vi "Ethernet IP Custom Device Initialization VI.vi"(8 "error in (no error)":errorcluster, 10 "Custom XML":string, 11 "Device Item Ref in":T1 format="%.0x") -> (0 "error out":errorcluster, 3 "Device Item Ref out":T1 format="%.0x")   [LabVIEW 2011, in "Ethernet IP Custom Device Custom Device.lvlib"]
uses:
  Ethernet IP Custom Device Custom Device.lvlib
  <vilib>/NI Veristand/Custom Device API/Custom Device Item Ref.ctl
  <vilib>/NI Veristand/Custom Device API/Custom Device Timed Loop Priority.ctl
  <vilib>/NI Veristand/Custom Device API/Custom Device Loop Type.ctl
  Ethernet IP Global Strings.vi
  Ethernet IP Global GUIDs.vi
  <vilib>/NI Veristand/Custom Device API/Set Item Property (String).vi
  <vilib>/NI Veristand/Custom Device API/Set Item Property (I32).vi
  <vilib>/NI Veristand/Custom Device API/Set Item Property (Path).vi
  <vilib>/NI Veristand/Custom Device API/Custom Device API.lvlib
panel:
  in  "Import Info":string="Unconfigured tags are tags that we need to specify if they are inputs or outputs.\n\nAlso provides information about tags that we couldn't import in a successful manner (due to incompatible data types for an example)."
  in  "IO Folder":string="Tags are devided up into an input section and an output section.\n \nPress the \"Input\" section in tree to see tag inputs and press the \"Output\"\nsection to see the tag outputs."
  in  "Description":string="This Custom Device will allow communication with targets that support communications using Logix tag names over Ethernet/IP.  \n\nValid targets include PLCs such as the Rockwell ControlLogix series.\n\nSupported data types in this custom device:\nSINT\nINT\nDINT\nREAL\nBOOL \nSTRING"
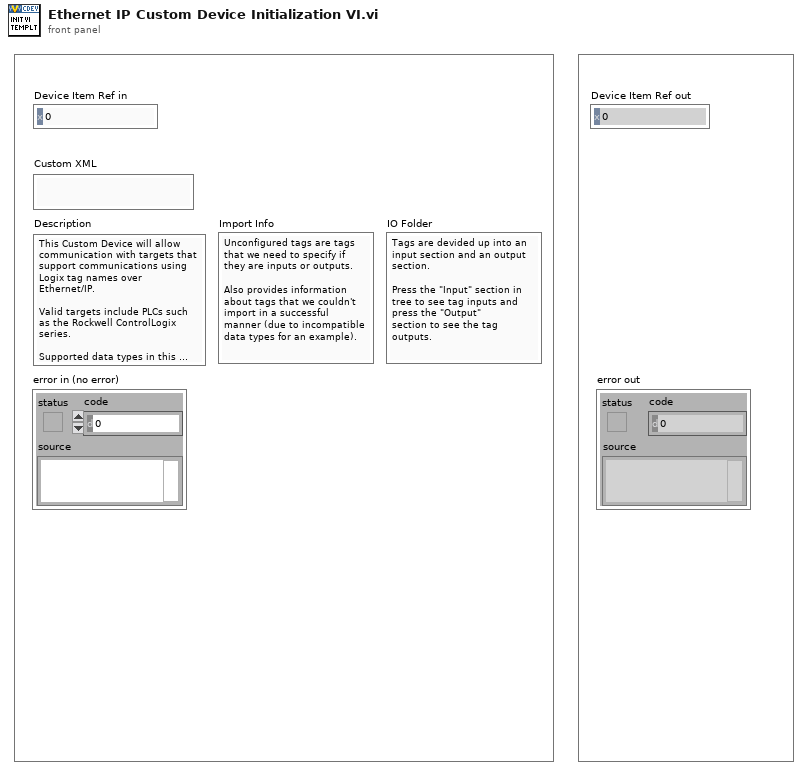
[diagram p1: front panel]
types:
  T1 = typedef "Custom Device API.lvlib/Custom Device Item Ref.ctl" = u64
  T2 = typedef "Custom Device API.lvlib/Custom Device Timed Loop Priority.ctl" = enum32{"Low", "Medium", "High"}
  T3 = typedef "Custom Device API.lvlib/Custom Device Loop Type.ctl" = enum32{"While Loop", "Timed Loop"}
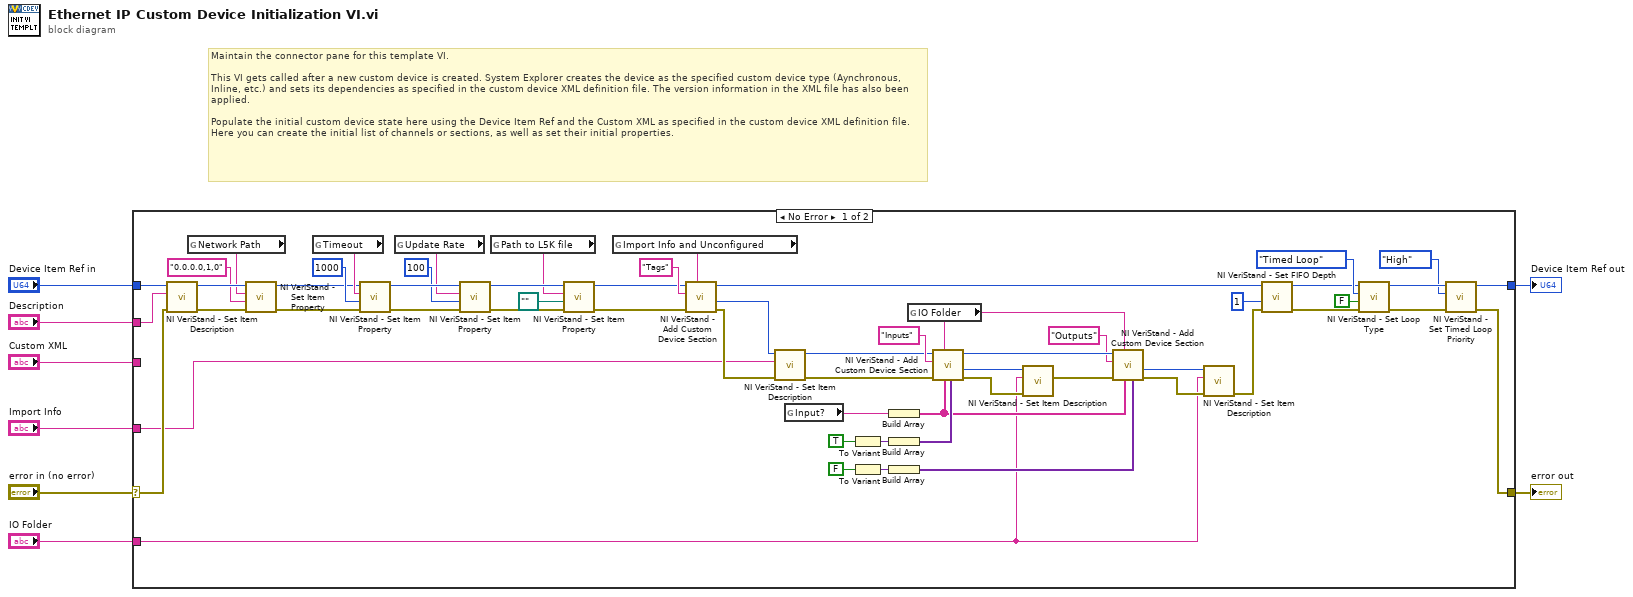
[diagram p0: block diagram]
diagram:
  # "Maintain the connector pane for this template VI.\n\nThis VI gets called after a new custom device is created. System Explorer creates the device as the specified custom device type (Aynchronous, Inline, etc.) and sets its dependencies as specified in the custom device XML definition file. The version information in the XML file has also been applied.\n\nPopulate the initial custom device state here using the Device Item Ref and the Custom XML as specified in the custom device XML definition file. Here you can create the initial list of channels or sections, as well as set their initial properties."
  n1 = case shown="No Error" "error in (no error)" {
    selector: "error in (no error)" -> [w58 w68]
    tunnel: [w9 w68] -> w8
    tunnel: [w12 w67] -> w6
    tunnel: "Device Item Ref in" -> [w63 w67]
    tunnel: "Custom XML" -> [_ _]
    tunnel: "Description" -> [w59 _]
    tunnel: "IO Folder" -> [w19 _]
    tunnel: "Import Info" -> [w18 _]
    frame No Error {
      n2 = call <vilib>:"NI VeriStand - Set Item Description.vi"("error in (no error)"=w58, "Description"=w59, "Item Ref in"=w63) -> ("error out"=w66:errorcluster, "Item Ref out"=w62:T1)  [unwired: 6 in, 1 out]
      n3 = global read "Ethernet IP Global Strings.vi" "Network Path"() -> (w57:string)
      n4 = call-poly <vilib>:"NI VeriStand - Set Item Property.vi"("error in (no error)"=w66, "Value"="0.0.0.0,1,0", "Property Name"=w57, "Item Ref in"=w62) -> ("error out"=w40:errorcluster, "Item Ref out"=w41:T1)  [unwired: 5 in, 1 out]
      n5 = global read "Ethernet IP Global Strings.vi" "Timeout"() -> (w56:string)
      n6 = call-poly <vilib>:"NI VeriStand - Set Item Property.vi"("error in (no error)"=w40, "Value"=1000, "Property Name"=w56, "Item Ref in"=w41) -> ("error out"=w64:errorcluster, "Item Ref out"=w61:T1)  [unwired: 5 in, 1 out]
      n7 = global read "Ethernet IP Global Strings.vi" "Update Rate"() -> (w55:string)
      n8 = call-poly <vilib>:"NI VeriStand - Set Item Property.vi"("error in (no error)"=w64, "Value"=100, "Property Name"=w55, "Item Ref in"=w61) -> ("error out"=w31:errorcluster, "Item Ref out"=w30:T1)  [unwired: 5 in, 1 out]
      n9 = global read "Ethernet IP Global Strings.vi" "Path to L5K file"() -> (w27:string)
      n10 = call-poly <vilib>:"NI VeriStand - Set Item Property.vi"("error in (no error)"=w31, "Value"=path "", "Property Name"=w27, "Item Ref in"=w30) -> ("error out"=w28:errorcluster, "Item Ref out"=w29:T1)  [unwired: 5 in, 1 out]
      n11 = global read "Ethernet IP Global GUIDs.vi" "Import Info and Unconfigured"() -> (w36:string)
      n12 = call <vilib>:"NI VeriStand - Add Custom Device Section.vi"("GUID (Default Section)"=w36, "error in (no error)"=w28, "Section Name"="Tags", "Parent Ref in"=w29) -> ("error out"=w34:errorcluster, "Section Ptr"=w35:T1, "Parent Ref out"=w37:T1)  [unwired: 4 in, 1 out]
      n13 = call <vilib>:"NI VeriStand - Set Item Description.vi"("error in (no error)"=w34, "Description"=w18, "Item Ref in"=w35) -> ("error out"=w33:errorcluster, "Item Ref out"=w32:T1)  [unwired: 6 in, 1 out]
      n14 = global read "Ethernet IP Global Strings.vi" "Input?"() -> (w42:string)
      n15 = To Variant(anything=TRUE) -> (Variant=w47:variant)
      n16 = To Variant(anything=FALSE) -> (Variant=w46:variant)
      n17 = Build Array(w42) -> (w43:string[])
      n18 = Build Array(w47) -> (w45:variant[])
      n19 = Build Array(w46) -> (w44:variant[])
      n20 = global read "Ethernet IP Global GUIDs.vi" "IO Folder"() -> (w50:string)
      n21 = call <vilib>:"NI VeriStand - Add Custom Device Section.vi"("Property Values"=w45, "Property names"=w43, "GUID (Default Section)"=w50, "error in (no error)"=w33, "Section Name"="Inputs", "Parent Ref in"=w32) -> ("error out"=w21:errorcluster, "Section Ptr"=w22:T1, "Parent Ref out"=w60:T1)  [unwired: 2 in, 1 out]
      n22 = call <vilib>:"NI VeriStand - Set Item Description.vi"("error in (no error)"=w21, "Description"=w19, "Item Ref in"=w22) -> ("error out"=w20:errorcluster)  [unwired: 6 in, 2 out]
      n23 = call <vilib>:"NI VeriStand - Add Custom Device Section.vi"("Property Values"=w44, "Property names"=w43, "GUID (Default Section)"=w50, "error in (no error)"=w20, "Section Name"="Outputs", "Parent Ref in"=w60) -> ("error out"=w24:errorcluster, "Section Ptr"=w25:T1)  [unwired: 2 in, 2 out]
      n24 = call <vilib>:"NI VeriStand - Set Item Description.vi"("error in (no error)"=w24, "Description"=w19, "Item Ref in"=w25) -> ("error out"=w23:errorcluster)  [unwired: 6 in, 2 out]
      n25 = call <vilib>:"NI VeriStand - Set FIFO Depth.vi"("error in (no error)"=w23, "Size FIFO Sink (1)"=u32 1 ("Size FIFO Source (1)"), "Device Ref in"=w37) -> ("error out"=w14:errorcluster, "Device Ref out"=w15:T1)  [unwired: 7 in]
      n26 = call <vilib>:"NI VeriStand - Set Loop Type.vi"("error in (no error)"=w14, "Use Device Clock (Timed Loops only)"=FALSE, "Loop type"=Custom_Device_Loop_Type."Timed Loop", "Device Ref in"=w15) -> ("error out"=w10:errorcluster, "Device Ref out"=w13:T1)  [unwired: 6 in]
      n27 = call <vilib>:"NI VeriStand - Set Timed Loop Priority.vi"("error in (no error)"=w10, "Priority"=Custom_Device_Timed_Loop_Priority."High", "Device Ref in"=w13) -> ("error out"=w9:errorcluster, "Device Ref out"=w12:T1)  [unwired: 7 in]
    }
    frame Error {
    }
  }
  "error out" <- w8
  "Device Item Ref out" <- w6
